vi "Get Topic.vi"(8 "error in (no error)":errorcluster, 9 "Topic Type":variant, 10 "Topic Name":string, 11 "TopicLookupTable":refnum<data-value>) -> (0 "error out":errorcluster, 2 "Topic Enqueuer":refnum<class "Message Enqueuer.lvclass">, 3 "TopicLookupTable":refnum<data-value>)   [LabVIEW 2017, in "Mediator.lvlib" / "TopicLookupTable.lvclass"]
doc: "<License>\nCopyright © 2017 Composed Systems, LLC | All rights reserved\nwww.composed.io\n\nAuthor: Ethan Stern <ethan.stern@composed.io>\n\nThis software is provided \"AS IS\" WITHOUT WARRANTIES, either express or implied, AND IS FOR EDUCATIONAL PURPOSES ONLY.\n</License>"
uses:
  TopicLookupTable.lvclass
  <vilib>/ActorFramework/Message Enqueuer/Message Enqueuer.lvclass
  TopicLookupTable.lvclass/TopicLookupTable.ctl
  <vilib>/ErrorRing/Error Ring.xnode
  <vilib>/Composed Systems/Variant Extensions/VariantExtensions.lvlib
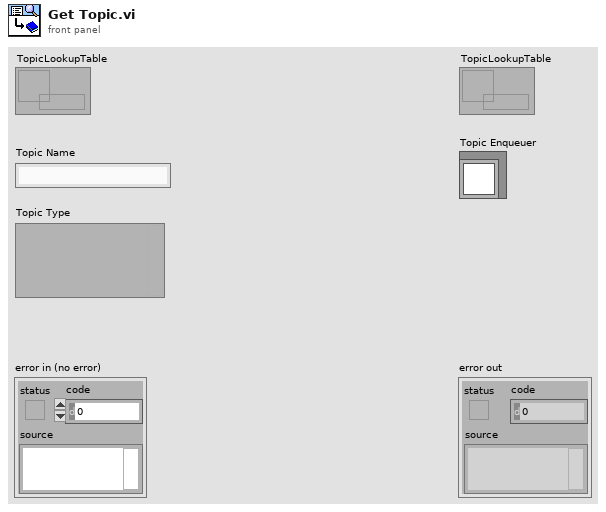
[diagram p1: front panel]
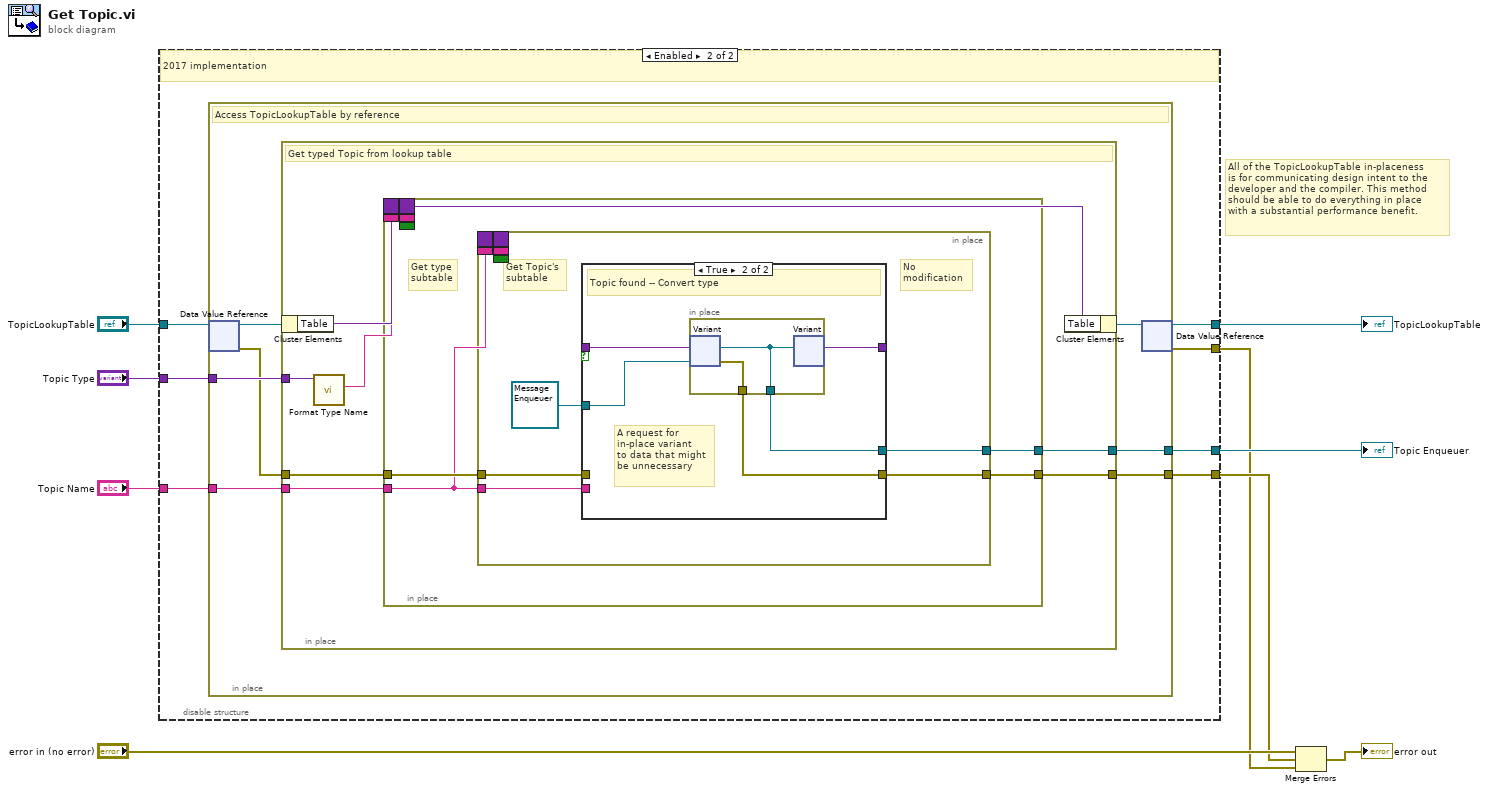
[diagram p0: block diagram]
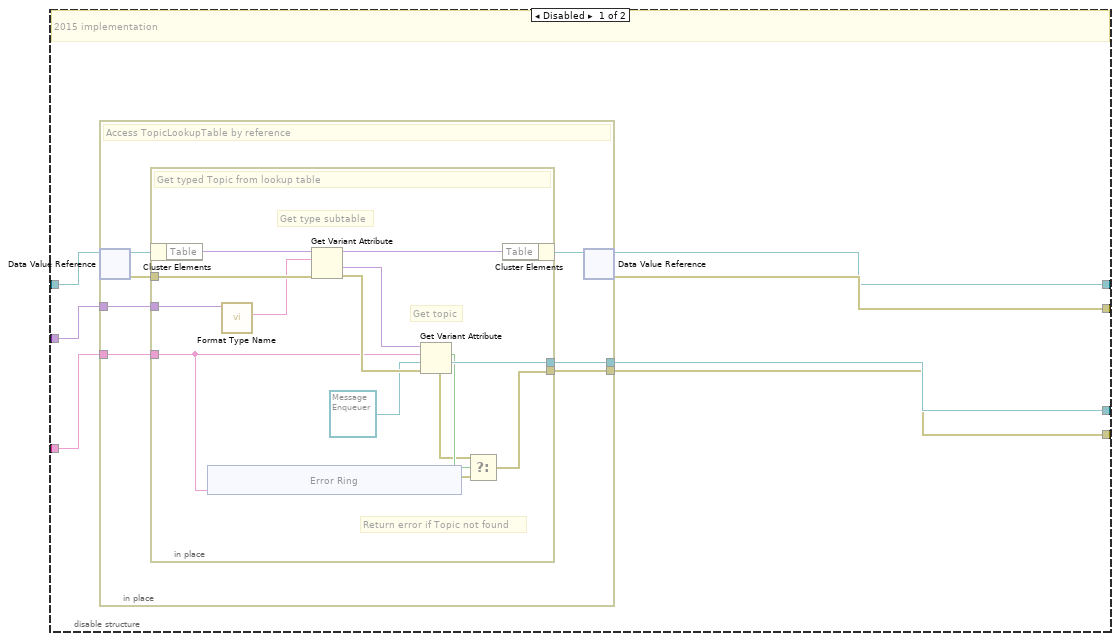
[diagram p2: hidden frame]
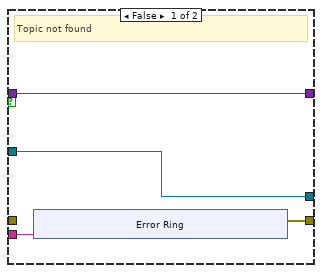
[diagram p3: hidden frame]
diagram:
  # "All of the TopicLookupTable in-placeness\nis for communicating design intent to the\ndeveloper and the compiler. This method\nshould be able to do everything in place\nwith a substantial performance benefit."
  n1 = disable-structure shown="Enabled" {
    disable-tunnel: "Topic Name" -> [w16 w49]
    disable-tunnel: "Topic Type" -> [w15 w48]
    disable-tunnel: [w14 w47] -> w5
    disable-tunnel: "TopicLookupTable" -> [w13 w46]
    disable-tunnel: [w12 w45] -> w3
    disable-tunnel: [w11 w44] -> w2
    disable-tunnel: [w10 w43] -> w1
    frame Disabled {
      # "2015 implementation"
      n2 = in-place {
        in-place-border: w16 -> [w23]
        in-place-border: w15 -> [w22]
        in-place-border: [w21] -> w12
        in-place-border: [w20] -> w14
        # "Access TopicLookupTable by reference"
        n3 = in-place-dvr #1(w13) -> (w19:refnum<class "TopicLookupTable.lvclass">, w17:errorcluster)
        n4 = in-place {
          in-place-border: w23 -> [w24]
          in-place-border: w22 -> [w32]
          in-place-border: [w31] -> w20
          in-place-border: [w26] -> w21
          in-place-border: w17 -> [w37]
          # "Return error if Topic not found"
          # "Get topic"
          # "Get type subtable"
          # "Get typed Topic from lookup table"
          n5 = in-place-cluster #2(w19) -> ("Table"=w36:variant)
          n6 = xnode "Error Ring"("parameter 0"=w24) -> ("error out"=w25:errorcluster)
          n7 = call <vilib>:"Format Type Name.vi"("Data Type"=w32) -> ("Type Name"=w33:string)  [unwired: 9 in, 1 out]
          n8 = Get Variant Attribute(Variant=w36, name=w33, error in=w37) -> (duplicate Variant=w34:variant, value=w35:variant, error out=w30:errorcluster)  [unwired: 1 in, 1 out]
          n9 = Get Variant Attribute(Variant=w35, name=w24, default value (empty Variant)=refnum<class "Message Enqueuer.lvclass"> refnum ("Self Enqueuer"), error in=w30) -> (found=w28:bool, value=w31:refnum<class "Message Enqueuer.lvclass">, error out=w27:errorcluster)  [unwired: 1 out]
          n10 = Select(t=w27, s=w28, f=w25) -> (s? t:f=w26:errorcluster)
          n11 = in-place-cluster #2("Table"=w34) -> (w18:refnum<class "TopicLookupTable.lvclass">)
        }
        n12 = in-place-dvr #1(w18) -> (w10:refnum<data-value>, w11:errorcluster)
      }
    }
    frame Enabled {
      # "2017 implementation"
      n13 = in-place {
        in-place-border: w49 -> [w56]
        in-place-border: w48 -> [w55]
        in-place-border: [w54] -> w45
        in-place-border: [w53] -> w47
        # "Access TopicLookupTable by reference"
        n14 = in-place-dvr #3(w46) -> (w52:refnum<class "TopicLookupTable.lvclass">, w50:errorcluster)
        n15 = in-place {
          in-place-border: w56 -> [w57]
          in-place-border: w55 -> [w60]
          in-place-border: [w63] -> w53
          in-place-border: [w62] -> w54
          in-place-border: w50 -> [w64]
          # "Get typed Topic from lookup table"
          n16 = in-place-cluster #4(w52) -> ("Table"=w61:variant)
          n17 = call <vilib>:"Format Type Name.vi"("Data Type"=w60) -> ("Type Name"=w59:string)  [unwired: 9 in, 1 out]
          n18 = in-place {
            in-place-border: w64 -> [w66]
            in-place-border: [w70] -> w63
            in-place-border: [w67] -> w62
            in-place-border: w57 -> [w65]
            border: w61 -> [_]
            border: w59 -> [_]
            border: [_] -> w58
            border: _ -> [_]
            border: _ -> [_]
            # "Get type\nsubtable"
            n19 = in-place {
              in-place-border: [w78] -> w70
              border: w69 -> [_]
              border: w65 -> [_]
              border: [_] -> w68
              border: _ -> [_]
              border: _ -> [_]
              in-place-border: w65 -> [w76]
              in-place-border: [w75] -> w67
              in-place-border: w66 -> [w74]
              # "No\nmodification"
              # "Get Topic's\nsubtable"
              n20 = case shown="True" w77 {
                tunnel: [w79 w88] -> w78
                tunnel: w76 -> [w82 _]
                tunnel: [w81 w90] -> w75
                tunnel: w74 -> [_ _]
                tunnel: w73 -> [w80 w92]
                tunnel: [w80 w91] -> w72
                tunnel: refnum<class "Message Enqueuer.lvclass"> refnum ("Self Enqueuer") -> [w79 w89]
                frame False {
                  # "Topic not found"
                  n21 = xnode "Error Ring"("parameter 0"=w82) -> ("error out"=w81:errorcluster)
                }
                frame True {
                  # "A request for\nin-place variant\nto data that might\nbe unnecessary"
                  # "Topic found -- Convert type"
                  n22 = in-place {
                    in-place-border: [w94] -> w88
                    in-place-border: [w93] -> w90
                    n23 = in-place-variant #5(w92, w89) -> (w94:refnum<class "Message Enqueuer.lvclass">, w93:errorcluster)
                    n24 = in-place-variant #5(w94) -> (w91:variant)  [unwired: 1 out]
                  }
                }
              }
            }
          }
          n25 = in-place-cluster #4("Table"=w58) -> (w51:refnum<class "TopicLookupTable.lvclass">)
        }
        n26 = in-place-dvr #3(w51) -> (w43:refnum<data-value>, w44:errorcluster)
      }
    }
  }
  "Topic Enqueuer" <- w5
  "TopicLookupTable" <- w1
  n27 = Merge Errors("error in (no error)", w3, w2) -> (→"error out":errorcluster)
